vi "Compare Value.vi"(8 "error in (no error)":errorcluster, 10 "new Value":variant, 11 "AISAS motor in":refnum<class "AISAS motor.lvclass">) -> (0 "error out":errorcluster, 1 "Motor Ok?":bool, 2 "same value?":bool, 3 "AISAS motor out":refnum<class "AISAS motor.lvclass">, 4 "new value":dbl, 6 "old value":dbl)   [LabVIEW 2014, in "AISAS motor.lvclass"]
uses:
  AISAS motor.lvclass
  AISAS motor.lvclass/AISAS motor.ctl
  Controls/Diffuser.ctl
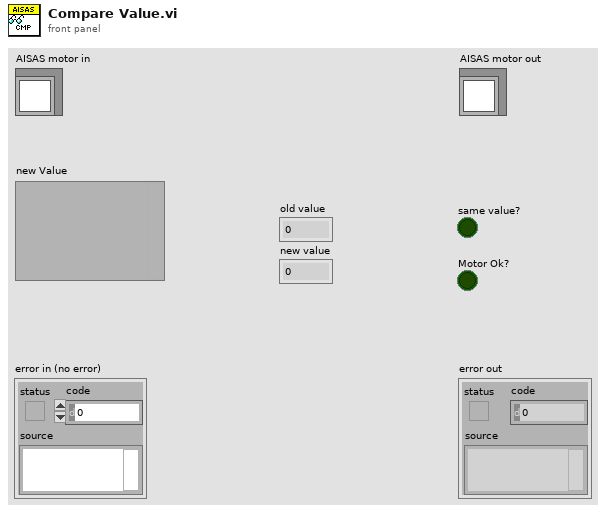
[diagram p1: front panel]
types:
  T1 = typedef "motor.ctl" = enum32{"Rotation", "Diffuser ", "Focus"}
  T2 = typedef "Diffuser.ctl" = enum16{"Out of Beam", "In Beam"}
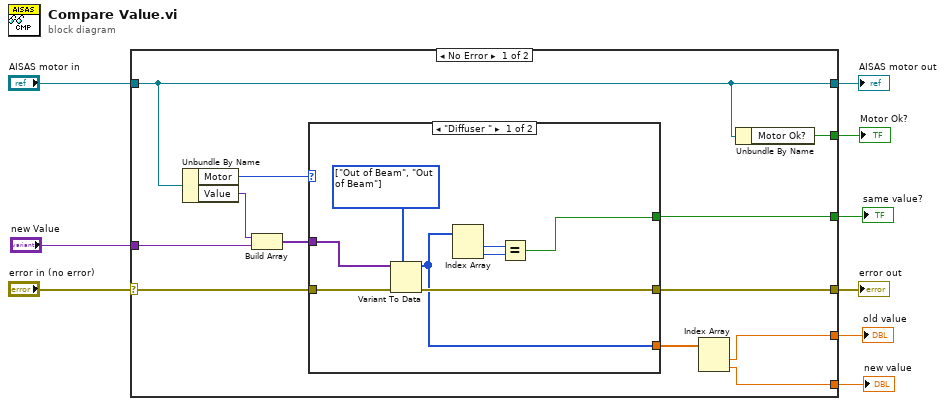
[diagram p0: block diagram]
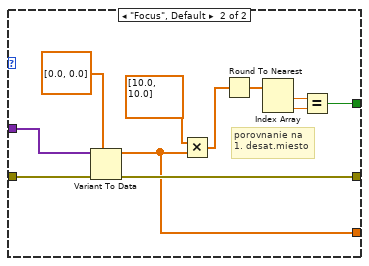
[diagram p2: hidden frame]
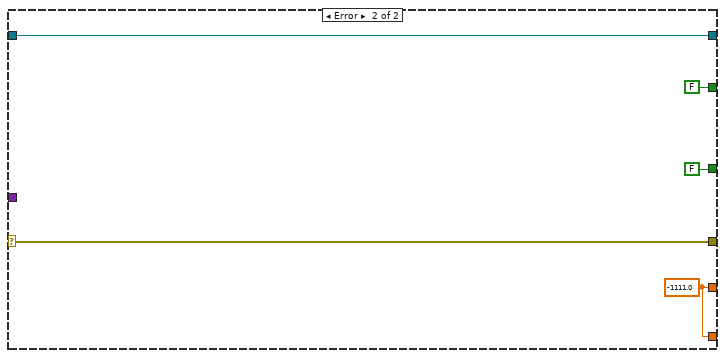
[diagram p3: hidden frame]
diagram:
  n1 = case shown="No Error" "error in (no error)" {
    selector: "error in (no error)" -> [w17 w44]
    tunnel: [w16 w44] -> w8
    tunnel: [w15 w45] -> w6
    tunnel: "AISAS motor in" -> [w15 w45]
    tunnel: "new Value" -> [w19 _]
    tunnel: [w14 FALSE ("Motor Ok?")] -> w4
    tunnel: [w13 FALSE] -> w3
    tunnel: [w11 w41] -> w2
    tunnel: [w10 w41] -> w1
    frame No Error {
      n2 = Unbundle By Name(w15) -> ("Motor"=w21:T1, "Value"=w20:variant)
      n3 = Build Array(w20, w19) -> (w18:variant[])
      n4 = case shown="\"Diffuser \"" w21 {
        tunnel: w18 -> [w29 w40]
        tunnel: w17 -> [w28 w39]
        tunnel: [w27 w38] -> w16
        tunnel: [w23 w31] -> w13
        tunnel: [w22 w30] -> w12
        frame "Diffuser " {
          w26 = T2[] [enum."Out of Beam", enum."Out of Beam"] items=["Out of Beam", "In Beam"]
          n5 = Variant To Data(error in=w28, type=w26, Variant=w29) -> (data=w22:T2[], error out=w27:errorcluster)
          n6 = Index Array(array=w22) -> (element #1=w25:T2, element #2=w24:T2)  [unwired: 2 in]
          n7 = Equal?(x=w25, y=w24) -> (x = y?=w23:bool)
        }
        frame "Focus", Default {
          # "porovnanie na\n1. desat.miesto"
          n8 = Variant To Data(error in=w39, type=dbl[] [0.0, 0.0], Variant=w40) -> (data=w30:dbl[], error out=w38:errorcluster)
          n9 = Multiply(x=dbl[] [10.0, 10.0], y=w30) -> (x*y=w36:dbl[])
          n10 = Round To Nearest(number=w36) -> (nearest integer value=w34:dbl[])
          n11 = Index Array(array=w34) -> (element #1=w32:dbl, element #2=w33:dbl)  [unwired: 2 in]
          n12 = Equal?(x=w32, y=w33) -> (x = y?=w31:bool)
        }
      }
      n13 = Index Array(array=w12) -> (element #1=w11:dbl, element #2=w10:dbl)  [unwired: 2 in]
      n14 = Unbundle By Name(w15) -> ("Motor Ok?"=w14:bool)
    }
    frame Error {
      w41 = -1111.0
    }
  }
  "error out" <- w8
  "AISAS motor out" <- w6
  "Motor Ok?" <- w4
  "same value?" <- w3
  "old value" <- w2
  "new value" <- w1
